vi "Print Report Dialog.vi"() -> (2 "Re-Print Current Report?":bool)   [LabVIEW 2010]
uses:
  _TypeDefs/OK Button_TouchScreen.ctl
panel:
  out "Message":string
  in  "Do Not Print":T1
  in  "Reprint Report?":T1
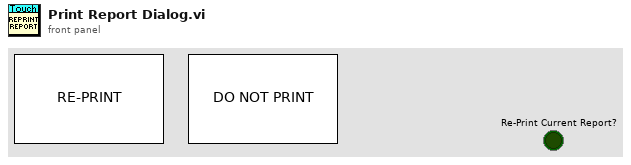
[diagram p1: front panel]
types:
  T1 = typedef "OK Button_TouchScreen.ctl" = bool
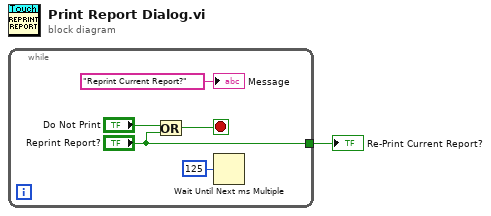
[diagram p0: block diagram]
diagram:
  n1 = while {
    tunnel: ["Reprint Report?"] -> w1
    stop <- w4 stop-if-true
    n2 = Or(x="Do Not Print", y="Reprint Report?") -> (x .or. y?=w4:T1)
    n3 = Wait Until Next ms Multiple(millisecond multiple=u32 125) -> ()  [unwired: 1 out]
    "Message" <- "Reprint Current Report?" ("Message")
  }
  "Re-Print Current Report?" <- w1
